vi "SMTP Email [NOOP].vi"(4 "error in (no error)":errorcluster, 7 "smtp session":T1) -> (0 "error out":errorcluster, 1 "reply":string, 2 "reply code":i32, 3 "smtp session out":T1)   [LabVIEW 2011, in "NewNI_SMTPEmail.lvlib"]
doc: "Sends the NOOP command to the SMTP server though connection specified as \"SMTP Session\", recieves reply and interprets it. This VI returns \"SMTP Session out.\" The results of the error interpretation go to the \"error out\" cluster."
uses:
  NewNI_SMTPEmail.lvlib
  SMTP Email Session.ctl
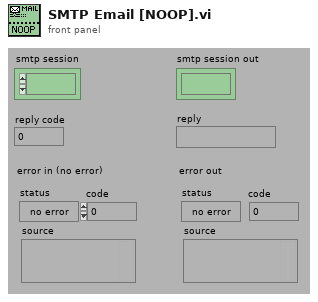
[diagram p1: front panel]
types:
  T1 = typedef "NewNI_SMTPEmail.lvlib/SMTP Email Session.ctl" = refnum<k1>
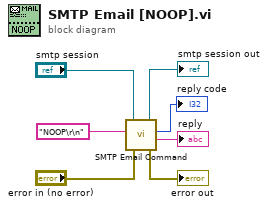
[diagram p0: block diagram]
diagram:
  n1 = call "SMTP Email Command.vi"("error in (no error)"="error in (no error)", "command"="NOOP\r\n" ("HELO"), "smtp session"="smtp session") -> ("error out"=→"error out":errorcluster, "reply"=→"reply":string, "reply code"=→"reply code":i32, "smtp session out"=→"smtp session out":T1)  [unwired: 1 out]
